vi "08_1.vi"() -> ()   [LabVIEW 2018]
uses:
  <userlib>/_OpenG.lib/array/array.llb/Remove Duplicates from 1D Array (I32)__ogtk.vi
panel:
  out "Numeric":i32
  in  "String":string
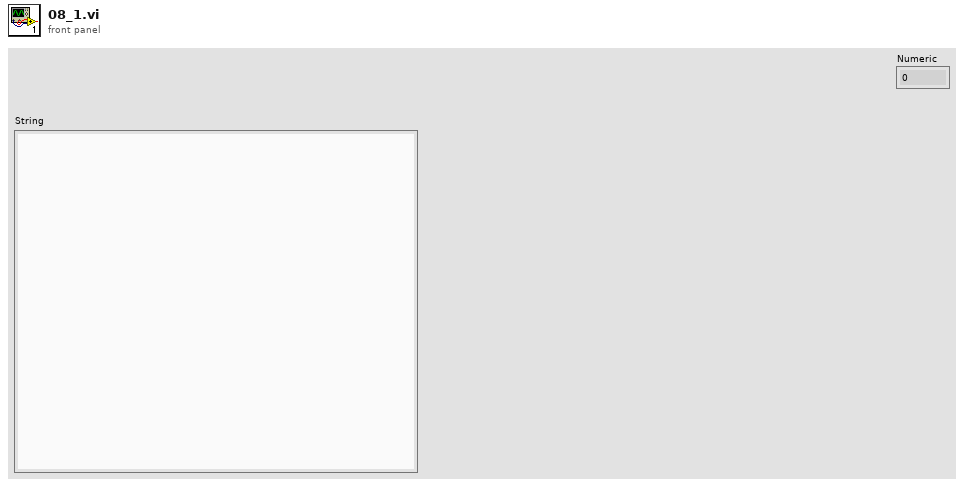
[diagram p1: front panel]
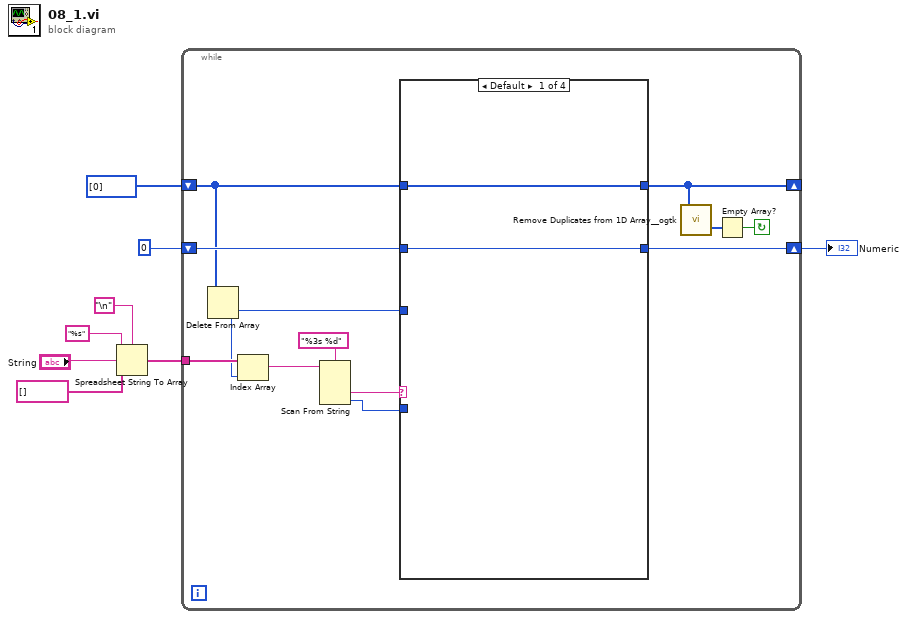
[diagram p0: block diagram]
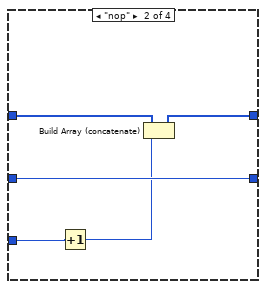
[diagram p2: hidden frame]
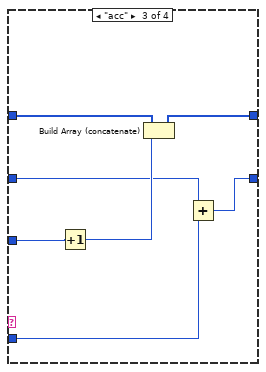
[diagram p3: hidden frame]
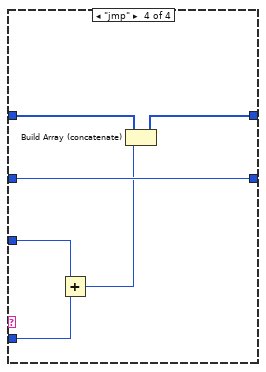
[diagram p4: hidden frame]
diagram:
  n1 = Spreadsheet String To Array(delimiter (Tab)="\n", format string="%s", spreadsheet string="String", array type (2D Dbl)=string[] []) -> (array=w4:string[])
  n2 = while {
    tunnel: w4 -> [w19]
    shift-right: [w15] -> w1
    shift-left: 0 -> [w16]
    shift-right: [w12] -> _
    shift-left: i32[] [0] -> [w13]
    stop <- w10 continue-if-true
    n3 = Delete From Array(array=w13) -> (deleted portion=w14:i32)  [unwired: 2 in, 1 out]
    n4 = Index Array(array=w19, index=w14) -> (element=w18:string)
    n5 = Scan From String(format string="%3s %d", input string=w18) -> (output 1=w17:string, output 2=w9:i32)  [unwired: 4 in, 3 out]
    n6 = case shown="Default" w17 {
      tunnel: w16 -> [w21 w27 w28 w40]
      tunnel: [w21 w27 w29 w40] -> w15
      tunnel: w14 -> [_ w26 w34 w38]
      tunnel: w13 -> [w22 w25 w33 w37]
      tunnel: [w22 w23 w31 w35] -> w12
      tunnel: w9 -> [_ _ w30 w39]
      frame Default {
      }
      frame "nop" {
        n7 = Increment(x=w26) -> (x+1=w24:i32)
        n8 = Build Array (concatenate)(w25, w24) -> (w23:i32[])
      }
      frame "acc" {
        n9 = Increment(x=w34) -> (x+1=w32:i32)
        n10 = Build Array (concatenate)(w33, w32) -> (w31:i32[])
        n11 = Add(x=w28, y=w30) -> (x+y=w29:i32)
      }
      frame "jmp" {
        n12 = Add(x=w38, y=w39) -> (x+y=w36:i32)
        n13 = Build Array (concatenate)(w37, w36) -> (w35:i32[])
      }
    }
    n14 = call-poly <userlib>:"Remove Duplicates from 1D Array__ogtk.vi"("Input Array"=w12) -> ("indices of removed elements"=w11:i32[])  [unwired: 1 out]
    n15 = Empty Array?(array=w11) -> (empty?=w10:bool)
  }
  "Numeric" <- w1
